vi "cDAQ UI - Handle Config Launch.vi"(8 "error in (no error)":errorcluster) -> (0 "error out":errorcluster, 2 "Not configured?":bool)   [LabVIEW 2011]
uses:
  Controls/INIT- READ - WRITE.ctl
  Controls/TransparencyEffectOperations.ctl
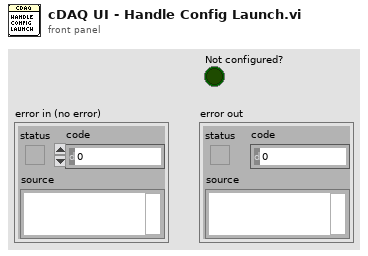
[diagram p1: front panel]
types:
  T1 = typedef "INIT- READ - WRITE.ctl" = enum16{"INIT", "READ", "WRITE"}
  T2 = typedef "TransparencyEffectOperations.ctl" = enum16{"Show", "Hide 80%", "Hide All"}
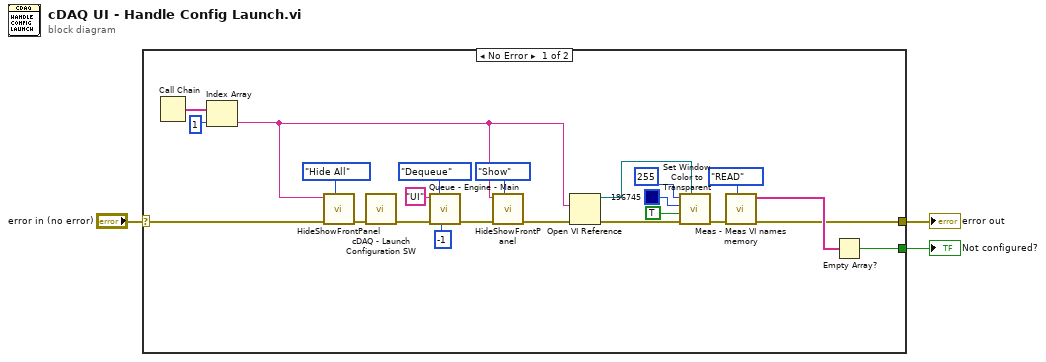
[diagram p0: block diagram]
diagram:
  n1 = case shown="No Error" "error in (no error)" {
    selector: "error in (no error)" -> [w15 w27]
    tunnel: [w5 w27] -> w3
    tunnel: [w4 _] -> w1
    frame No Error {
      n2 = Call Chain() -> (call chain=w14:string[])
      n3 = Index Array(array=w14, index=1) -> (element=w10:string)
      n4 = call "HideShowFrontPanel.vi"("Operation"=TransparencyEffectOperations."Hide All", "Error In"=w15, "VI Name Or Path (Caller)"=w10) -> ("Error Out"=w20:errorcluster)  [unwired: 8 in]
      n5 = call "cDAQ - Launch Configuration SW.vi"("error in"=w20) -> ("error out"=w19:errorcluster)  [unwired: 10 in]
      n6 = call "Queue - Engine - Main.vi"("timeout in ms (-1)"=-1, "Operation"=enum16{"Enqueue", "Dequeue", "Flush", "Release"}."Dequeue", "error in"=w19, "Queue Name In"="UI") -> ("error out"=w22:errorcluster)  [unwired: 5 in, 2 out]
      n7 = call "HideShowFrontPanel.vi"("Operation"=TransparencyEffectOperations."Show", "Error In"=w22, "VI Name Or Path (Caller)"=w10) -> ("Error Out"=w12:errorcluster)  [unwired: 8 in]
      n8 = Open VI Reference(vi path=w10, error in (no error)=w12) -> (vi reference=w9:refnum<vi>, error out=w11:errorcluster)  [unwired: 4 in]
      n9 = call "Set Window Color to Transparent.vi"("Calling VI's reference"=w9, "error in (no error)"=w11, "Activate"=TRUE, "Color to Replace"=u32 196745, "Factor"=u8 255) -> ("error out"=w8:errorcluster)  [unwired: 3 in]
      n10 = call "Meas - Meas VI names memory.vi"("Operation"=INIT-_READ_-_WRITE."READ", "Error In"=w8) -> ("Error Out"=w5:errorcluster, "Names Out"=w6:string[])  [unwired: 8 in]
      n11 = Empty Array?(array=w6) -> (empty?=w4:bool)
    }
    frame Error {
    }
  }
  "error out" <- w3
  "Not configured?" <- w1
